vi "Swerve_Module CanCoder_Set Status Periods.vi"(6 "TimeoutMs":u32=300, 7 "Max # Of Tries":i32=5, 8 "Error":errorcluster, 11 "CTRE_CANcoder_DeviceRef":T1) -> (0 "Error Out":errorcluster, 3 "CTRE_CANcoder_DeviceRef Out":T1)   [LabVIEW 2020]
uses:
  <vilib>/Rock Robotics/WPI/ThirdParty/Phoenix-LabVIEW/CANCoder/Controls/CTRE_Phoenix_CANcoder_DeviceRef.ctl
  <vilib>/Rock Robotics/WPI/ThirdParty/Phoenix-LabVIEW/CANCoder/Controls/CTRE_Phoenix_CANcoder_StatusFrame.ctl
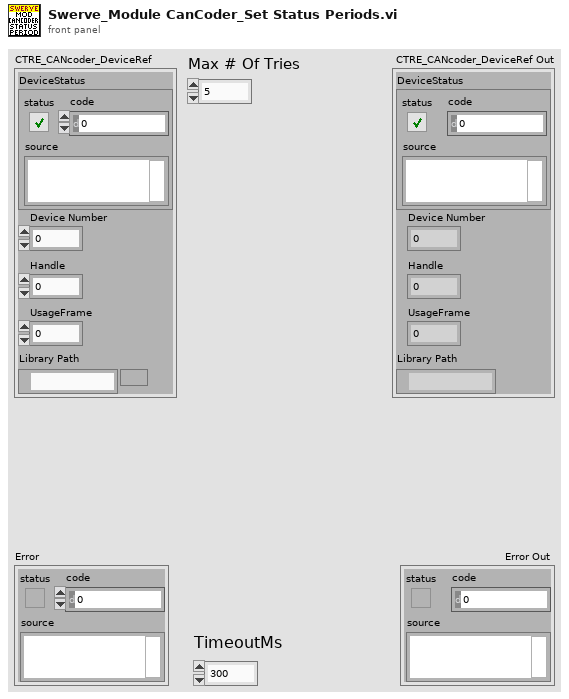
[diagram p1: front panel]
types:
  T1 = typedef "CTRE_Phoenix_CANcoder_DeviceRef.ctl" = cluster{"DeviceStatus":errorcluster, "Device Number":u8, "Handle":u64, "UsageFrame":u32, "Library Path":path}
  T2 = typedef "CTRE_Phoenix_CANcoder_StatusFrame.ctl" = u32
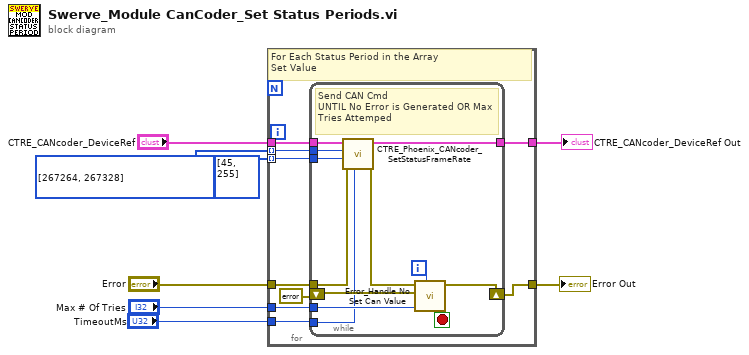
[diagram p0: block diagram]
diagram:
  w5 = T2[] [267264, 267328] items=["SensorData"=267264, "VbatAndFaults"=267328] ("Array")
  n1 = for {
    tunnel: "CTRE_CANcoder_DeviceRef" -> [w16]
    tunnel: w5 -> [w13] mode=indexing
    tunnel: "Error" -> [w14]
    tunnel: [w17] -> w6
    tunnel: [w15] -> w3
    tunnel: "Max # Of Tries" -> [w11]
    tunnel: "TimeoutMs" -> [w10]
    tunnel: u8[] [45, 255] ("Period (ms)") -> [w9] mode=indexing
    # "For Each Status Period in the Array\nSet Value"
    n2 = while {
      tunnel: w16 -> [w24]
      tunnel: w13 -> [w18]
      tunnel: w14 -> [w22]
      tunnel: [w23] -> w15
      shift-right: [w29] -> w17
      shift-left: errorcluster {"status"=FALSE, "code"=0, "source"=""} ("Error Out") -> [w26]
      tunnel: w11 -> [w25]
      tunnel: w10 -> [w20]
      tunnel: w9 -> [w19]
      i -> [w27]
      stop <- w28 stop-if-true
      # "Send CAN Cmd\nUNTIL No Error is Generated OR Max Tries Attemped"
      n3 = call <vilib>:"CTRE_Phoenix_CANcoder_SetStatusFrameRate.vi"("timeoutMs"=w20, "error in (no error)"=w22, "Period (ms)"=w19, "CANcoder Status Frame"=w18, "CTRE_CANcoder_DeviceRef"=w24) -> ("error out"=w21:errorcluster, "CTRE_CANcoder_DeviceRef"=w23:T1)  [unwired: 5 in]
      n4 = call "Error_Handle No Set Can Value.vi"("Max # Of Tries"=w25, "Loop Itteration"=w27, "Previous Error"=w26, "Error"=w21) -> ("Stop Out"=w28:bool, "Error Out"=w29:errorcluster)  [unwired: 6 in]
    }
  }
  "Error Out" <- w6
  "CTRE_CANcoder_DeviceRef Out" <- w3
